vi "Axis_Home FGV.vi"(7 "Enum":enum16{"Initial", "write", "read"}(ring)=enum."read", 9 "Home":bool, 10 "Axis":i32) -> (1 "HMStatus":bool, 2 "HMSStatus":bool[](array[boolean]))   [LabVIEW 2019]
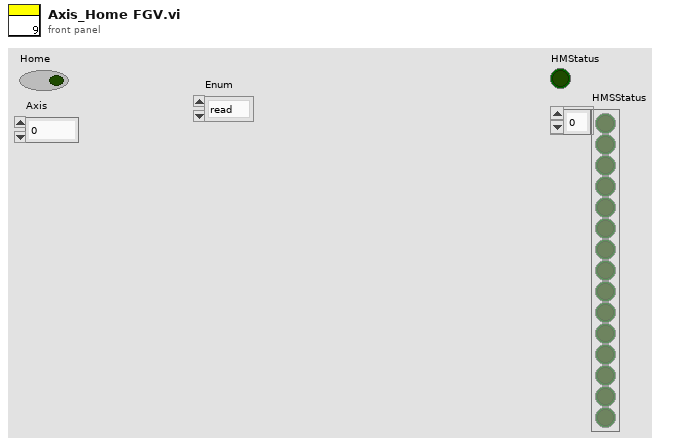
[diagram p1: front panel]
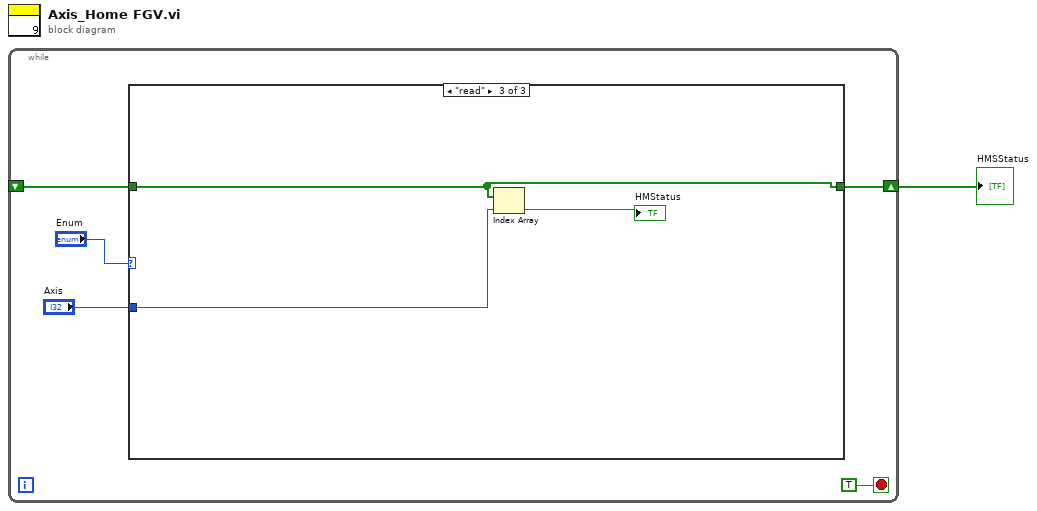
[diagram p0: block diagram]
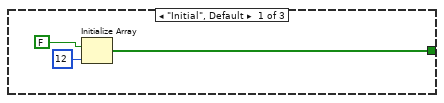
[diagram p2: hidden frame]
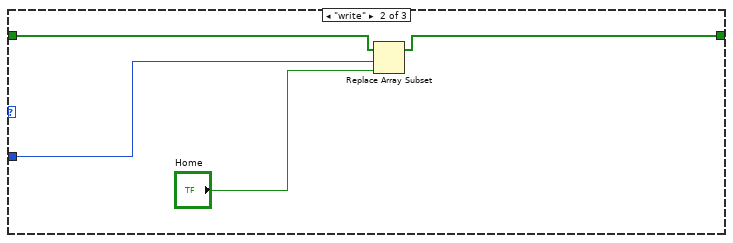
[diagram p3: hidden frame]
diagram:
  n1 = while {
    shift-right: [w5] -> w1
    shift-left: _ -> [w4]
    stop <- TRUE stop-if-true
    n2 = case shown="\"read\"" "Enum" {
      tunnel: [w7 w12 w16] -> w5
      tunnel: w4 -> [_ w13 w16]
      tunnel: "Axis" -> [_ w10 w15]
      frame "Initial", Default {
        n3 = Initialize Array(FALSE, 12 ("dimension size")) -> (w7:bool[])
      }
      frame "write" {
        n4 = Replace Array Subset(array=w13, new element="Home", index=w10) -> (w12:bool[])
      }
      frame "read" {
        n5 = Index Array(array=w16, index=w15) -> (element=→"HMStatus":bool)
      }
    }
  }
  "HMSStatus" <- w1
